vi "项解析.vi"(11 "配置信息":T2) -> (3 "任务列表解析":cluster{"启用":bool, "任务":T1[]})   [LabVIEW 2022 SP3, in "Cleaning cycle.lvclass"]
uses:
  Cleaning cycle.lvclass
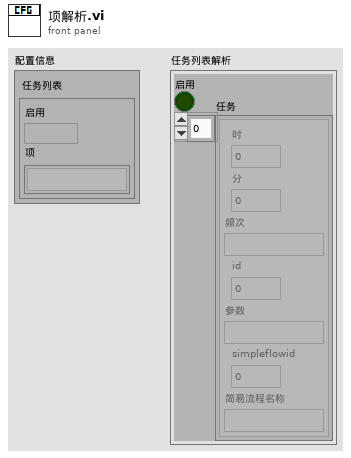
[diagram p1: front panel]
types:
  T1 = typedef "Cleaning cycle.lvclass/周期项.ctl" = cluster{"时":i32, "分":i32, "频次":string, "id":i32, "参数":string, "simpleflowid":i32, "简易流程名称":string}
  T2 = typedef "Cleaning cycle.lvclass/配置信息.ctl" = cluster{"任务列表":T3}
  T3 = typedef "Cleaning cycle.lvclass/任务.ctl" = cluster{"启用":bool, "项":string[][]}
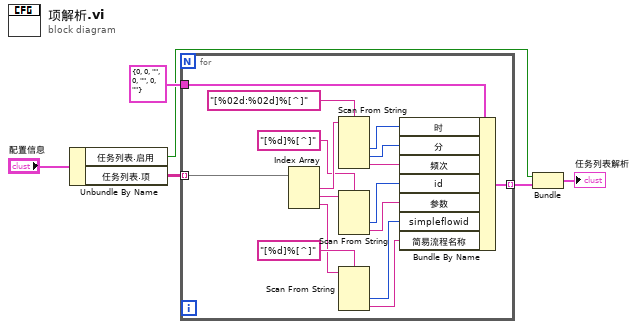
[diagram p0: block diagram]
diagram:
  n1 = Unbundle By Name("配置信息") -> ("任务列表.启用"=w2:bool, "任务列表.项"=w4:string[][])
  n2 = for {
    tunnel: w4 -> [w22] mode=indexing
    tunnel: T1 {"时"=0, "分"=0, "频次"="", "id"=0, "参数"="", "simpleflowid"=0, "简易流程名称"=""} ("周期项") -> [w15]
    tunnel: [w7] -> w3 mode=indexing
    n3 = Index Array(array=w22) -> (element #1=w20:string, element #2=w17:string, element #3=w16:string)  [unwired: 3 in]
    n4 = Scan From String(format string="[%02d:%02d]%[^]" ("格式字符串"), input string=w20) -> (output 1=w14:i32, output 2=w13:i32, output 3=w12:string)  [unwired: 5 in, 3 out]
    n5 = Scan From String(format string="[%d]%[^]" ("格式字符串"), input string=w17) -> (output 1=w11:i32, output 2=w10:string)  [unwired: 4 in, 3 out]
    n6 = Scan From String(format string="[%d]%[^]" ("格式字符串"), input string=w16) -> (output 1=w9:i32, output 2=w8:string)  [unwired: 4 in, 3 out]
    n7 = Bundle By Name(cluster=w15, "时"=w14, "分"=w13, "频次"=w12, "id"=w11, "参数"=w10, "simpleflowid"=w9, "简易流程名称"=w8) -> (w7:T1)
  }
  n8 = Bundle("启用"=w2, w3) -> (→"任务列表解析":cluster{"启用":bool, T1[]})  [unwired: 1 in]
